vi "Analog Output - 1 Channel - N Samples.vi"() -> ()   [LabVIEW 2019]
uses:
  <vilib>/myRIO/Common/Instrument Driver Framework/ELVIS III v1.0/AO Block/vis/ELVIS III v1.0 Close AO Block.vi
  <vilib>/myRIO/Common/Instrument Driver Framework/myRIO v1.0/UART/vis/myRIO v1.0 Close UART.vi
  <vilib>/myRIO/Common/Instrument Driver Framework/ELVIS III v1.0/AO Block/vis/ELVIS III v1.0 Unreserve AO Block.vi
  <vilib>/myRIO/Common/Instrument Driver Framework/ELVIS III v1.0/AO Block/vis/ELVIS III v1.0 Build MUX Configuration AO Block.vi
  <vilib>/Utility/error.llb/Error Cluster From Error Code.vi
  <vilib>/myRIO/Common/Instrument Driver Framework/ELVIS III v1.0/AO Block/vis/ELVIS III v1.0 AO Block Write.vi
  <vilib>/myRIO/Common/Instrument Driver Framework/ELVIS III v1.0/Resource Manager/vis/ELVIS III v1.0 Unreserve Channel List.vi
  <vilib>/myRIO/Common/Instrument Driver Framework/myRIO v1.0/myRIO v1.0 Close.vi
  <vilib>/myRIO/Common/Instrument Driver Framework/Utilities/vis/FPGA Ref Manager.vi
  <vilib>/myRIO/Common/Instrument Driver Framework/ELVIS III v1.0/ELVIS III v1.0 Reset FPGA.vi
  <vilib>/myRIO/Common/Instrument Driver Framework/myRIO v1.0/IRQ/vis/myRIO v1.0 IRQ Info FGV.vi
  <vilib>/myRIO/Common/Instrument Driver Framework/myRIO v1.0/IRQ/vis/myRIO v1.0 Timer IRQ Info FGV.vi
  <vilib>/myRIO/Common/Instrument Driver Framework/myRIO v1.0/IRQ/vis/myRIO v1.0 ISR Agent.vi
  <vilib>/myRIO/Instrument Drivers/Utilities/vis/Reset Index.vi
  <vilib>/myRIO/Common/Instrument Driver Framework/myRIO v1.0/Resource Manager/vis/myRIO v1.0 Block Write Resource Manager.vi
  <vilib>/myRIO/Instrument Drivers/Utilities/Utilities.lvlib
  <vilib>/myRIO/Instrument Drivers/Onboard IO/AO Block/AO Block.lvlib
panel:
  in  "Generate Waveform":bool
  in  "Frequency (Hz)":dbl=10.0 format="%#_13g"
  in  "Amplitude (V)":dbl=5.0 min=-10.0 max=10.0 step=0.1 format="%#_13g"
  in  "Stop":bool
  # "ELVIS III Control IO"
  # "模拟输出单通道"
  # "Overview: Generates one period of a sine wave on Bank A, Channel AO0 (A/AO0).\nInstructions:\n1. Configure the sine wave properties below.\n2. Connect A/AO0 to the positive lead of the load, and connect AGND to the negative lead of the load. AGND is the ground reference terminal for analog output channels.\n3. Run the VI.\n4. Press Generate Waveform to output the sine wave on A/AO0."
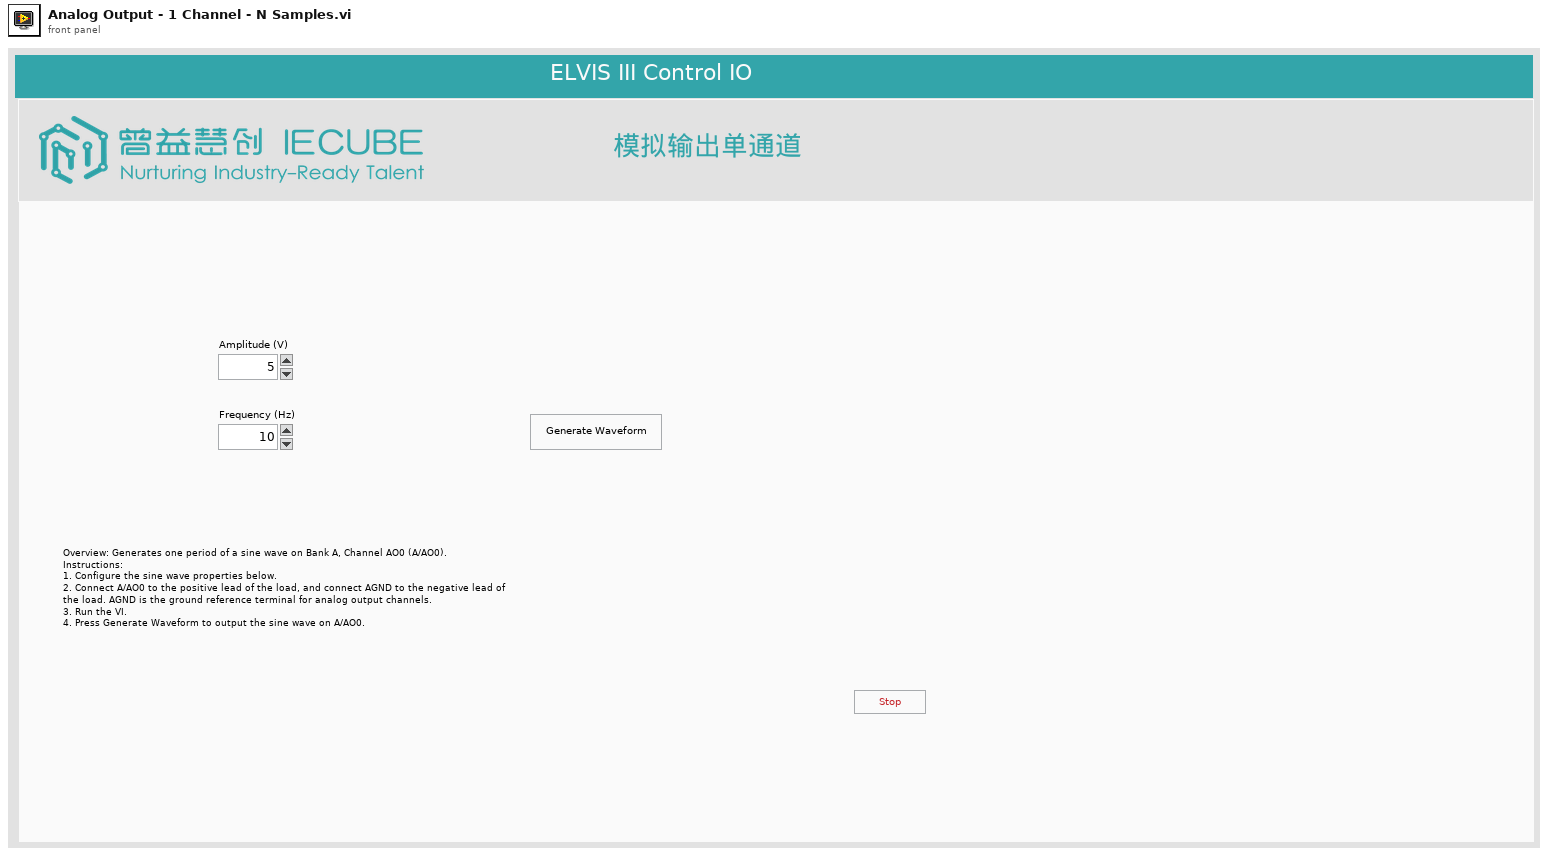
[diagram p1: front panel]
types:
  T1 = typedef "AO Block.lvlib/AO Block Reference.ctl" = cluster{"myRIO Reference":T2, "AO (N Samples) Channels List":T6, "AO (N Samples) Scaling Constants List":T8[]}
  T2 = typedef "myRIO Generic Hardware Reference.ctl" = cluster{"myRIO Model":T3, "myRIO Hardware Reference":T4}
  T3 = typedef "Hardware Version Enum.ctl" = enum16{"Unknown", "myRIO-1900", "myRIO-1950", "roboRIO", "NI ELVIS RIO CM", "ELVIS III"}
  T4 = typedef "myRIO v1.0 Reference.ctl" = cluster{"Generic FPGA Reference":T5, "Allow multiple opens":bool}
  T5 = typedef "Generic FPGA Reference.ctl" = refnum<k20>
  T6 = typedef "AO Block Channels List.ctl" = T7[]
  T7 = typedef "AO Block Channels Enum.ctl" = enum16{"Not Connected", "A/AO0 (N Samples)", "A/AO1 (N Samples)", "B/AO0 (N Samples)", "B/AO1 (N Samples)"}
  T8 = typedef "Analog Scaling Constants.ctl" = cluster{"LSB Weight (Volts)":dbl, "Offset (Volts)":dbl, "Signed?":bool}
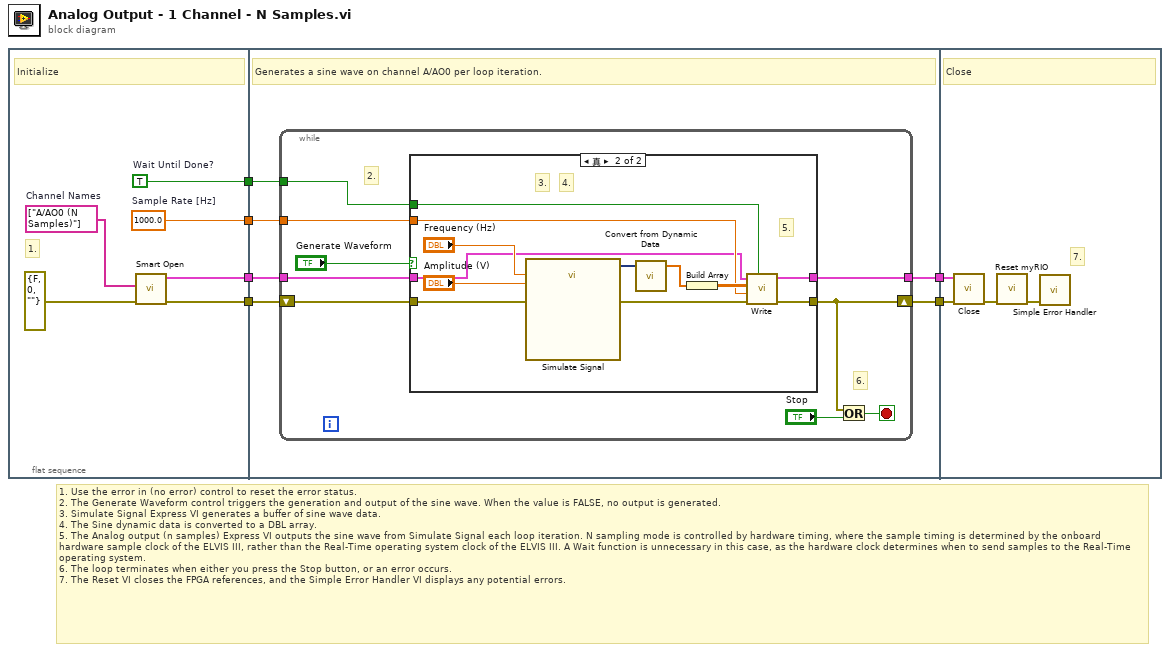
[diagram p0: block diagram]
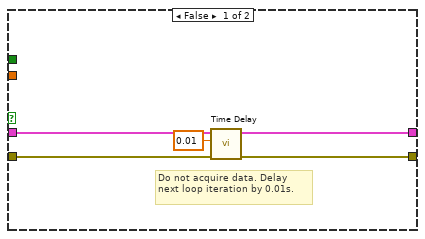
[diagram p2: hidden frame]
diagram:
  # "1. Use the error in (no error) control to reset the error status. \n2. The Generate Waveform control triggers the generation and output of the sine wave. When the value is FALSE, no output is generated.\n3. Simulate Signal Express VI generates a buffer of sine wave data.\n4. The Sine dynamic data is converted to a DBL array.\n5. The Analog output (n samples) Express VI outputs the sine wave from Simulate Signal each loop iteration. N sampling mode is controlled by hardware timing, where the sample timing is determined by the onboard hardware sample clock of the ELVIS III, rather than the Real-Time operating system clock of the ELVIS III. A Wait function is unnecessary in this case, as the hardware clock determines when to send samples to the Real-Time operating system.\n6. The loop terminates when either you press the Stop button, or an error occurs.\n7. The Reset VI closes the FPGA references, and the Simple Error Handler VI displays any potential errors."
  n1 = flat-sequence {
    tunnel: [w11] -> w5
    tunnel: [w9] -> w4
    tunnel: [w8] -> w3
    tunnel: [w7] -> w1
    tunnel: [w18] -> w6
    tunnel: w5 -> [w17]
    tunnel: w4 -> [w16]
    tunnel: w3 -> [w15]
    tunnel: [w14] -> w2
    tunnel: w1 -> [w13]
    tunnel: w6 -> [w45]
    tunnel: w2 -> [w44]
    frame #0 {
      w9 = TRUE  # Wait Until Done?
      w8 = 1000.0  # Sample Rate [Hz]
      w12 = tag[] ["A/AO0 (N Samples)"]  # Channel Names
      # "1."
      # "Initialize"
      n2 = call <vilib>:"Smart Open.vi"("error in (no error)"=errorcluster {"status"=FALSE, "code"=0, "source"=""} ("Error In"), "Channel Names"=w12) -> ("error out"=w11:errorcluster, "AO (N Samples) Ref Out"=w7:T1)  [unwired: 8 in]
    }
    frame #1 {
      # "Generates a sine wave on channel A/AO0 per loop iteration."
      n3 = while {
        shift-right: [w26] -> w18
        shift-left: w17 -> [w25]
        tunnel: w16 -> [w22]
        tunnel: w15 -> [w21]
        tunnel: [w20] -> w14
        tunnel: w13 -> [w19]
        stop <- w27 stop-if-true
        # "6."
        # "2."
        n4 = case shown="真" "Generate Waveform" {
          tunnel: [w30 w37] -> w26
          tunnel: w25 -> [w29 w43]
          tunnel: w22 -> [_ w35]
          tunnel: w21 -> [_ w34]
          tunnel: [w28 w33] -> w20
          tunnel: w19 -> [w28 w32]
          frame False {
            # "Do not acquire data. Delay next loop iteration by 0.01s."
            n5 = call "Time Delay"("error in (no error)"=w29, "Delay Time (s)"=0.01) -> ("error out"=w30:errorcluster)  [unwired: 9 in]
          }
          frame True {
            # "5."
            # "4."
            # "3."
            n6 = call "Simulate Signal"("Frequency"="Frequency (Hz)", "Amplitude"="Amplitude (V)", "error in (no error)"=w43) -> ("Sine"=w40:dynamicdata, "error out"=w36:errorcluster)  [unwired: 11 in]
            n7 = call "Convert from Dynamic Data"("Dynamic Data Type"=w40) -> ("Array"=w38:dbl[])  [unwired: 3 in]
            n8 = Build Array(w38) -> (w39:dbl[][])
            n9 = call <vilib>:"Write.vi"("Wait Until Done?"=w35, "error in (no error)"=w36, "Sample Rate [Hz]"=w34, "Values"=w39, "AO (N Samples) Ref In"=w32) -> ("error out"=w37:errorcluster, "AO (N Samples) Ref Out"=w33:T1)  [unwired: 5 in]
          }
        }
        n10 = Or(x=w26, y="Stop") -> (x .or. y?=w27:bool)
      }
    }
    frame #2 {
      # "7."
      # "Close"
      n11 = call <vilib>:"Close.vi"("error in (no error)"=w45, "AO (N Samples) Ref In"=w44) -> ("error out"=w46:errorcluster)  [unwired: 9 in]
      n12 = call <vilib>:"Reset myRIO.vi"("error in (no error)"=w46) -> ("error out"=w47:errorcluster)  [unwired: 10 in]
      n13 = call <vilib>:"Simple Error Handler.vi"("error in (no error)"=w47) -> ()  [unwired: 4 in, 5 out]
    }
  }
